vi "去除均值.vi"(11 "输入信号":dbl[](array[numeric])) -> (3 "去均值信号":dbl[](array[numeric]))   [LabVIEW 2014]
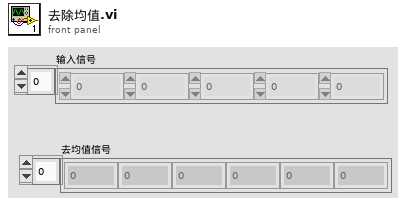
[diagram p1: front panel]
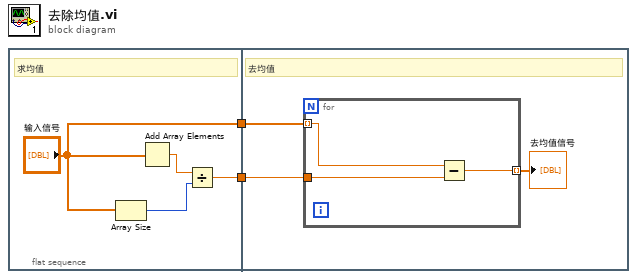
[diagram p0: block diagram]
diagram:
  n1 = flat-sequence "平铺式顺序结构" {
    tunnel: ["输入信号"] -> w2
    tunnel: [w3] -> w1
    tunnel: w2 -> [w9]
    tunnel: w1 -> [w8]
    frame #0 {
      # "求均值"
      n2 = Array Size(array="输入信号") -> (size(s)=w5:i32)
      n3 = Add Array Elements(numeric array="输入信号") -> (sum=w6:dbl)
      n4 = Divide(x=w6, y=w5) -> (x/y=w3:dbl)
    }
    frame #1 {
      # "去均值"
      n5 = for {
        tunnel: w9 -> [w12] mode=indexing
        tunnel: w8 -> [w11]
        tunnel: [w10] -> w7 mode=indexing
        n6 = Subtract(x=w12, y=w11) -> (x-y=w10:dbl)
      }
      "去均值信号" <- w7
    }
  }
